vi "AD5781WriteRead.vi"(8 "Write":u32 format="%032b") -> (0 "WriteEqualsRead":bool, 3 "Readback":u32 format="%032b")   [LabVIEW 2014]
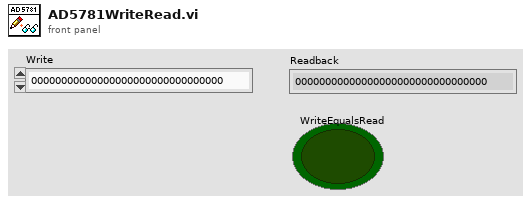
[diagram p1: front panel]
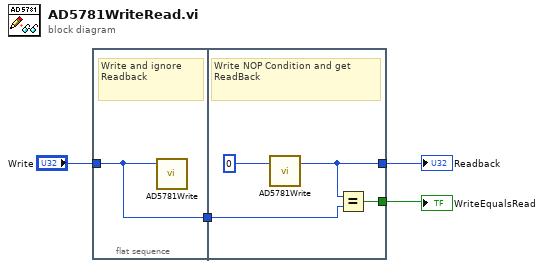
[diagram p0: block diagram]
diagram:
  n1 = flat-sequence {
    tunnel: "Write" -> [w5]
    tunnel: [w5] -> w2
    tunnel: [w8] -> w3
    tunnel: w2 -> [w7]
    tunnel: [w6] -> w1
    frame #0 {
      # "Write and ignore Readback"
      n2 = call "AD5781Write.vi"("U32"=w5) -> ()  [unwired: 3 in, 1 out]
    }
    frame #1 {
      # "Write NOP Condition and get ReadBack"
      n3 = call "AD5781Write.vi"("U32"=u32 0) -> ("Readback"=w8:u32)  [unwired: 3 in]
      n4 = Equal?(x=w8, y=w7) -> (x = y?=w6:bool)
    }
  }
  "Readback" <- w3
  "WriteEqualsRead" <- w1
